vi "GetNISeq.vi"(0 "Pre-Looks":i32, 1 "Type of scan":u16=1, 3 "NI Card":refnum<k15>, 7 "errorin":errorcluster, 8 "File Array":string[](array[string]), 9 "Divide prf by":i32, 10 "lines per plane":i32, 11 "Channel (0)":i32, 12 "Start Record":i32, 14 "save?":bool=TRUE, 15 "Reverse?":bool) -> ()   [LabVIEW 2022 SP3]
uses:
  Motion Controllers/-MotionRoutines/MotionGlobals.vi
  Acqiris/-AcqirisRoutines/VScaleInfoAcq.vi
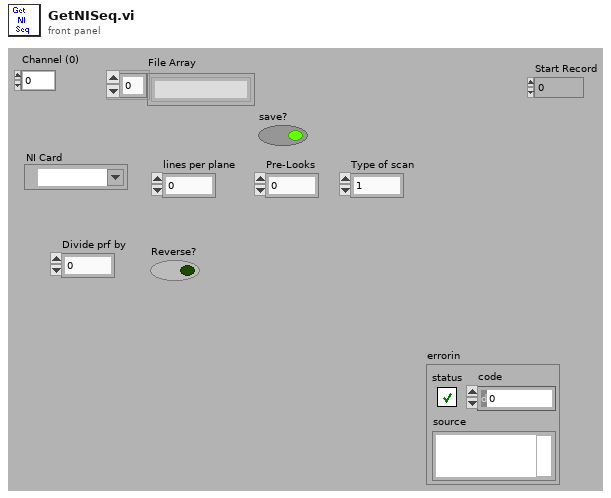
[diagram p1: front panel]
types:
  T1 = cluster{sgl, "Gain [dB]  ":sgl, "Atten (dB)":sgl}
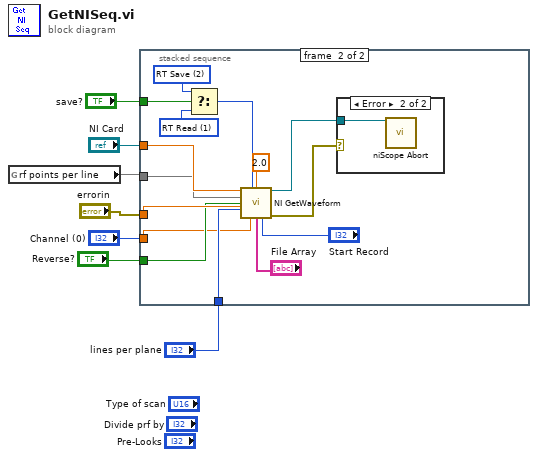
[diagram p0: block diagram]
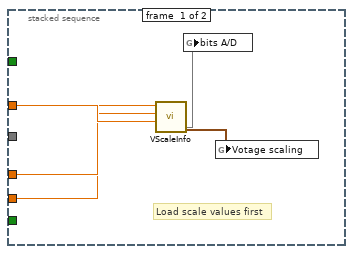
[diagram p2: hidden frame]
diagram:
  n1 = global read "MotionGlobals.vi" "rf points per line"() -> (w4)
  n2 = stacked-sequence {
    tunnel: w4 -> [_ w17]
    tunnel: "lines per plane" -> [_ w27]
    tunnel: "errorin" -> [w10 w26]
    tunnel: "Reverse?" -> [_ w24]
    tunnel: "NI Card" -> [w12 w22]
    tunnel: "Channel (0)" -> [w8 w23]
    tunnel: "save?" -> [_ w21]
    frame #0 {
      # "Load scale values first"
      n3 = call-poly "VScaleInfo.vi"() -> (4:w9, "vGain scalar"=w8:dbl, "vGain (dB)"=w10:dbl, "Total Gain (dB)"=w12:dbl, "Voltage Scale"=w11:T1)  [unwired: 6 in]
      n4 = global write "MotionGlobals.vi" "bits A/D"(w9) -> ()
      n5 = global write "MotionGlobals.vi" "Votage scaling"(w11) -> ()
    }
    frame #1 {
      w18 = u16 2 items=["Simple Read", "RT Read", "RT Save", "Scaled Voltage"] ("Read Method")
      w19 = u16 1 items=["Simple Read", "RT Read", "RT Save", "Scaled Voltage"] ("Read Method")
      n6 = Select(t=w18, s=w21, f=w19) -> (s? t:f=w20:u16)
      n7 = call "NI GetWaveform.vi"("Acq ID In"=w22, "Read Method"=w20, "timeout"=2.0, "Num Samps"=w17, "Reverse?"=w24, "Num Segs"=w27, "error in"=w26, "Channel"=w23, "File Array"="File Array", "Start Record"="Start Record") -> ("Acq ID Out"=w14:refnum<k15>, "error out"=w15:errorcluster)  [unwired: 4 out]
      n8 = case shown="Error" w15 {
        tunnel: w14 -> [_ w28]
        frame No Error {
        }
        frame Error {
          n9 = call <instrlib>:"niScope Abort.vi"("instrument handle"=w28) -> ()  [unwired: 1 in, 14 out]
        }
      }
    }
  }
